vi "LensMotor_init.vi"(7 "modIdTag":string="S1", 8 "error in (no error)":errorcluster, 10 "position":sgl, 11 "channel":refnum<k24>) -> (0 "error out":errorcluster)   [LabVIEW 2021]
uses:
  D:/psychometric_function_v2/lib/Grpc.Core.dll
  lib/Grpc.Core.dll
  D:/psychometric_function_v2/lib/FossilProtosSharp.dll
  lib/FossilProtosSharp.dll
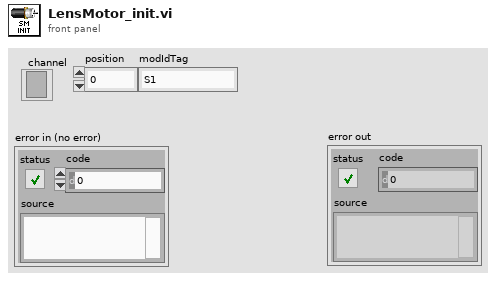
[diagram p1: front panel]
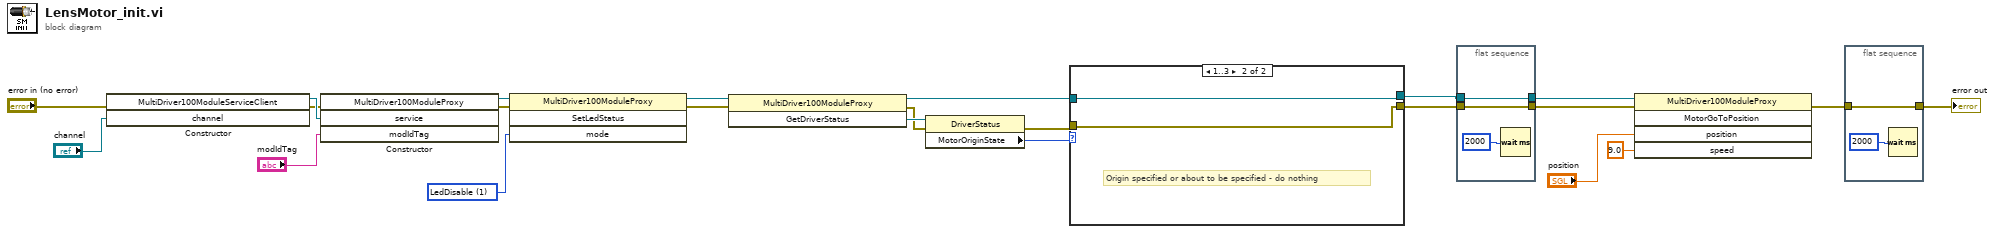
[diagram p0: block diagram]
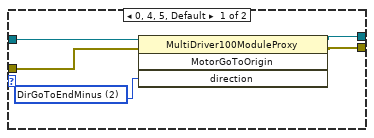
[diagram p2: hidden frame]
diagram:
  w18 = 1 items=["LedUnspecified", "LedDisable", "LedEnable", "LedOnlyErrors", "LedStatus"] ("mode")
  n1 = constructor class="MultiDriver100ModuleServiceClie"(error in="error in (no error)", "channel"="channel") -> (reference out=w17:refnum<k24>, error out=w16:errorcluster)  [unwired: 2 in, 2 out]
  n2 = constructor class="MultiDriver100ModuleProxy"(error in=w16, "service"=w17, "modIdTag"="modIdTag") -> (reference out=w20:refnum<k24>, error out=w19:errorcluster)  [unwired: 2 in, 3 out]
  n3 = invoke class="MultiDriver100ModuleProxy" method="SetLedStatus"(reference=w20, error in=w19, "mode"=w18) -> (reference out=w4:refnum<k24>, error out=w3:errorcluster)  [unwired: 1 in, 2 out]
  n4 = invoke class="MultiDriver100ModuleProxy" method="GetDriverStatus"(reference=w4, error in=w3) -> (reference out=w5:refnum<k24>, error out=w8:errorcluster, "GetDriverStatus"=w9:refnum<k24>)  [unwired: 1 in]
  n5 = property class="DriverStatus"(reference=w9, error in=w8) -> (error out=w6:errorcluster, "MotorOriginState"=w7:i32)  [unwired: 1 out]
  n6 = case shown="1..3" w7 {
    tunnel: w6 -> [w27 w29]
    tunnel: w5 -> [w26 w30]
    tunnel: [w25 w29] -> w1
    tunnel: [w24 w30] -> w2
    frame 0, 4, 5, Default {
      w28 = 2 items=["DirUnspecified", "DirGoToEndPlus", "DirGoToEndMinus"] ("direction")
      n7 = invoke class="MultiDriver100ModuleProxy" method="MotorGoToOrigin"(reference=w26, error in=w27, "direction"=w28) -> (reference out=w24:refnum<k24>, error out=w25:errorcluster)  [unwired: 1 in, 2 out]
    }
    frame 1..3 {
      # "Origin specified or about to be specified - do nothing"
    }
  }
  n8 = flat-sequence {
    tunnel: w1 -> [w33]
    tunnel: [w33] -> w13
    tunnel: w2 -> [w32]
    tunnel: [w32] -> w12
    frame #0 {
      n9 = Wait (ms)(milliseconds to wait=u32 2000) -> ()  [unwired: 1 out]
    }
  }
  n10 = invoke class="MultiDriver100ModuleProxy" method="MotorGoToPosition"(reference=w12, error in=w13, "position"="position", "speed"=sgl 9.0) -> (error out=w11:errorcluster)  [unwired: 1 in, 4 out]
  n11 = flat-sequence {
    tunnel: w11 -> [w35]
    tunnel: [w35] -> w10
    frame #0 {
      n12 = Wait (ms)(milliseconds to wait=u32 2000) -> ()  [unwired: 1 out]
    }
  }
  "error out" <- w10
